vi "example_wait_for_value_change_1.vi"() -> ()   [LabVIEW 2015]
panel:
  in  "Boolean 3":bool
  in  "Time Stamp":timestamp
  in  "Numeric":dbl
  in  "Meter":dbl(knob) scale=0.0..10.0
  in  "String":string
  in  "Boolean 2":bool
  in  "Boolean":bool
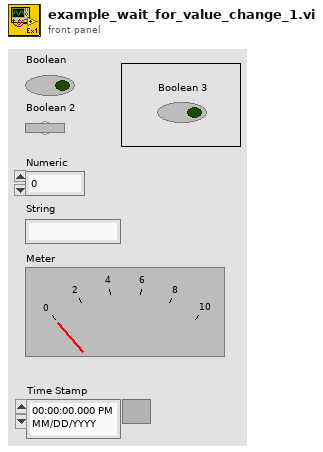
[diagram p1: front panel]
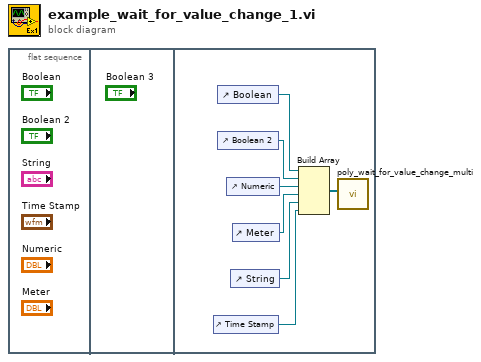
[diagram p0: block diagram]
diagram:
  n1 = flat-sequence {
    frame #0 {
    }
    frame #1 {
    }
    frame #2 {
      n2 = control-ref of="Time Stamp"() -> (w7:refnum<vi>)
      n3 = control-ref of="Boolean"() -> (w1:refnum<vi>)
      n4 = control-ref of="Boolean 2"() -> (w2:refnum<vi>)
      n5 = control-ref of="Numeric"() -> (w4:refnum<vi>)
      n6 = control-ref of="String"() -> (w6:refnum<vi>)
      n7 = control-ref of="Meter"() -> (w5:refnum<vi>)
      n8 = Build Array(w1, w2, w4, w5, w6, w7) -> (w3:refnum<vi>[])
      n9 = call "poly_wait_for_value_change_multi.vi"("control ref"=w3) -> ()  [unwired: 10 in, 1 out]
    }
  }
